vi "VI Tree.vi"   [LabVIEW 2012, in "Phidget Frequency Counter.lvlib"]
doc: "${FrequencyCounter:VITreeHeader}"
uses:
  <instrlib>/Phidgets/Phidget Frequency Counter/Phidget Frequency Counter.lvlib
  <instrlib>/Phidgets/Phidget Frequency Counter/Public/FrequencyCounterStart.vi
  <instrlib>/Phidgets/Phidget Frequency Counter/Public/FrequencyCounterOpen.vi
  <instrlib>/Phidgets/Phidget Frequency Counter/Public/FrequencyCounterClose.vi
panel:
  # "(c) 2015 Phidgets Inc..  ALL RIGHTS RESERVED."
  # "SEE DIAGRAM\nFOR VI TREE."
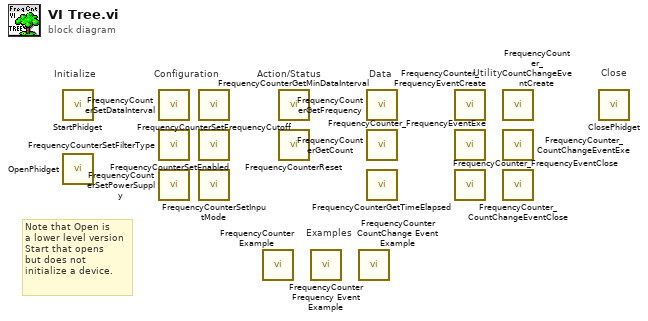
[diagram p0: block diagram]
diagram:
  # "Note that Open is\na lower level version\nStart that opens\nbut does not \ninitialize a device."
  # "Examples"
  # "Configuration"
  # "Utility"
  # "Data"
  # "Action/Status"
  # "Close"
  # "Initialize"
  n1 = call-poly <instrlib>:"StartPhidget.vi"() -> ()  [unwired: 12 in, 4 out]
  n2 = call-poly <instrlib>:"OpenPhidget.vi"() -> ()  [unwired: 8 in, 4 out]
  n3 = call <instrlib>:"FrequencyCounterSetDataInterval.vi"() -> ()  [unwired: 9 in, 2 out]
  n4 = call <instrlib>:"FrequencyCounterSetFilterType.vi"() -> ()  [unwired: 9 in, 2 out]
  n5 = call <instrlib>:"FrequencyCounterSetPowerSupply.vi"() -> ()  [unwired: 9 in, 2 out]
  n6 = call <instrlib>:"FrequencyCounterSetFrequencyCutoff.vi"() -> ()  [unwired: 9 in, 2 out]
  n7 = call <instrlib>:"FrequencyCounterSetEnabled.vi"() -> ()  [unwired: 9 in, 2 out]
  n8 = call <instrlib>:"FrequencyCounterSetInputMode.vi"() -> ()  [unwired: 9 in, 2 out]
  n9 = call <instrlib>:"FrequencyCounter Example.vi"() -> ()  [unwired: 12 in]
  n10 = call <instrlib>:"FrequencyCounterGetMinDataInterval.vi"() -> ()  [unwired: 8 in, 3 out]
  n11 = call <instrlib>:"FrequencyCounterReset.vi"() -> ()  [unwired: 9 in, 2 out]
  n12 = call <instrlib>:"FrequencyCounter Frequency Event Example.vi"() -> ()  [unwired: 12 in]
  n13 = call <instrlib>:"FrequencyCounter CountChange Event Example.vi"() -> ()  [unwired: 12 in]
  n14 = call <instrlib>:"FrequencyCounterGetFrequency.vi"() -> ()  [unwired: 8 in, 3 out]
  n15 = call <instrlib>:"FrequencyCounterGetCount.vi"() -> ()  [unwired: 8 in, 3 out]
  n16 = call <instrlib>:"FrequencyCounterGetTimeElapsed.vi"() -> ()  [unwired: 8 in, 3 out]
  n17 = call <instrlib>:"FrequencyCounter_FrequencyEventCreate.vi"() -> ()  [unwired: 9 in, 3 out]
  n18 = call <instrlib>:"FrequencyCounter_FrequencyEventExe.vi"() -> ()  [unwired: 5 in, 7 out]
  n19 = call <instrlib>:"FrequencyCounter_FrequencyEventClose.vi"() -> ()  [unwired: 10 in, 2 out]
  n20 = call <instrlib>:"FrequencyCounter_CountChangeEventCreate.vi"() -> ()  [unwired: 9 in, 3 out]
  n21 = call <instrlib>:"FrequencyCounter_CountChangeEventExe.vi"() -> ()  [unwired: 8 in, 8 out]
  n22 = call <instrlib>:"FrequencyCounter_CountChangeEventClose.vi"() -> ()  [unwired: 10 in, 2 out]
  n23 = call-poly <instrlib>:"ClosePhidget.vi"() -> ()  [unwired: 11 in, 1 out]
